vi "Insert CRC.vi"(8 "error in (no error)":errorcluster, 9 "Recalculate CRC?":bool, 10 "Frame Infos":T1 {"CRC Index" min=-7 max=7; "DLC Length  Corruption Index" min=-8 max=8}, 11 "CAN frame in":T3 {"payload" format="%x"; "timestamp" format="%<%.7X\n%x>T"; "type" items=["CAN Data"=0, "CAN Remote"=1, "CAN Bus Error"=2, "CAN 2.0 Data"=8, "CAN FD Data"=16, "CAN FD+BRS Data"=24, "J1939 Data"=192, "Delay"=224, "Log Trigger"=225, "Start Trigger"=226]; "identifier" format="%x"}) -> (0 "error out":errorcluster, 3 "CAN frame out":T3 {"payload" format="%x"; "timestamp" format="%<%.7X\n%x>T"; "type" items=["CAN Data"=0, "CAN Remote"=1, "CAN Bus Error"=2, "CAN 2.0 Data"=8, "CAN FD Data"=16, "CAN FD+BRS Data"=24, "J1939 Data"=192, "Delay"=224, "Log Trigger"=225, "Start Trigger"=226]; "identifier" format="%x"})   [LabVIEW 2018, in "CAN Gateway Engine.lvlib"]
uses:
  CAN Gateway Engine.lvlib
  <vilib>/xnet/xnet.llb/XNET Frame CAN.ctl
  <vilib>/xnet/xnet.llb/XNET Frame Type CAN.ctl
  Shared/CTLs/Frame.ctl
  Shared/CTLs/Signal_Data_Trigger.ctl
  Shared/CAN Gateway Shared.lvlib
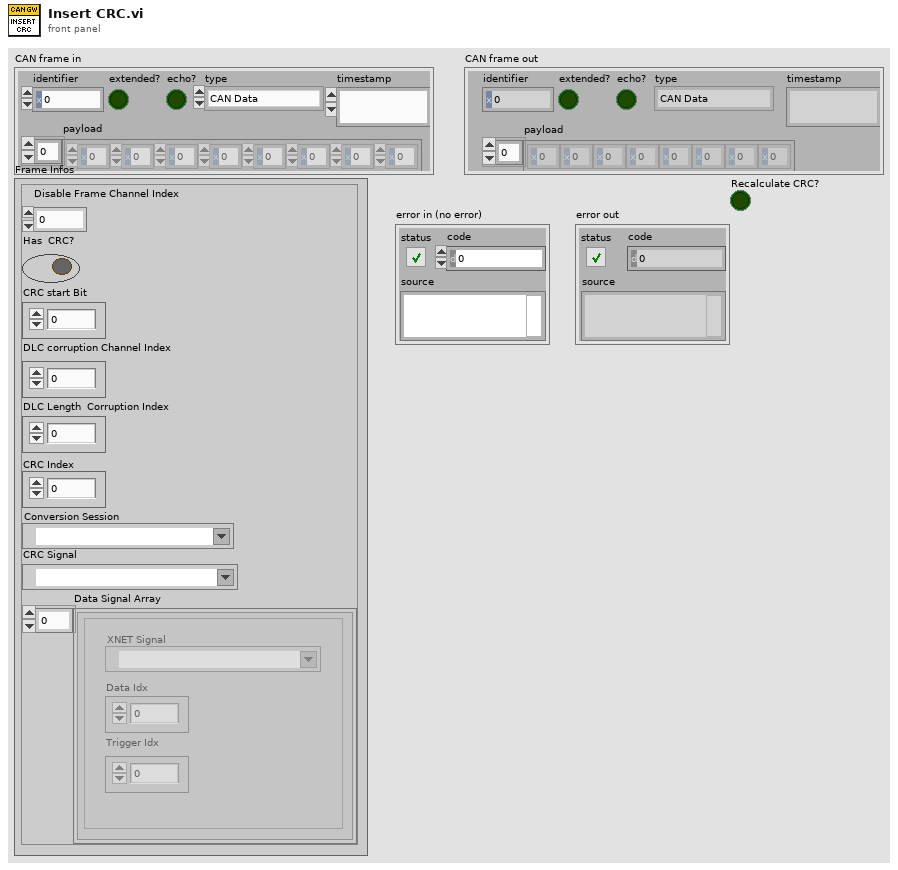
[diagram p1: front panel]
types:
  T1 = typedef "CAN Gateway Shared.lvlib/Frame.ctl" = cluster{"Disable Frame Channel Index":i32, "Has  CRC?":bool, "CRC start Bit":u32, "DLC corruption Channel Index":i32, "DLC Length  Corruption Index":i32, "CRC Index":i32, "Conversion Session":refnum<k21>, "CRC Signal":refnum<k21>, "Data Signal Array":T2[]}
  T2 = typedef "CAN Gateway Shared.lvlib/Signal_Data_Trigger.ctl" = cluster{"XNET Signal":refnum<k21>, "Data Idx":u32, "Trigger Idx":u32}
  T3 = typedef "XNET Frame CAN.ctl" = cluster{"timestamp":timestamp, "payload":u8[], "identifier":u32, "type":T4, "extended?":bool, "echo?":bool}
  T4 = typedef "XNET Frame Type CAN.ctl" = u8
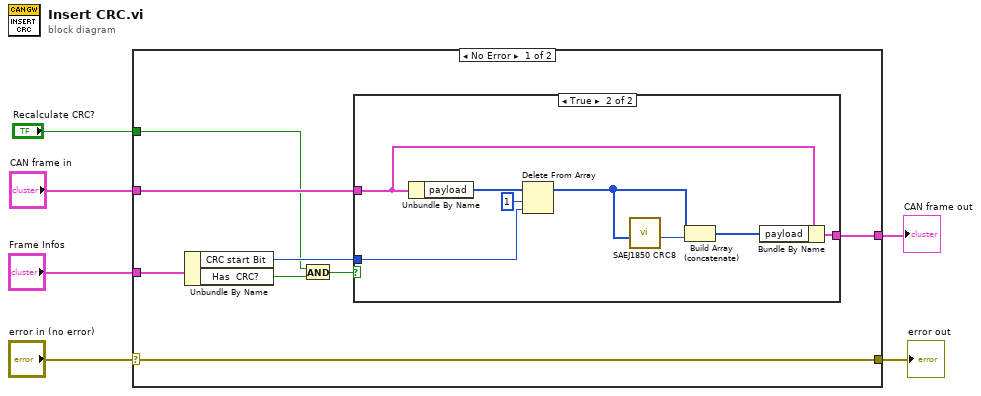
[diagram p0: block diagram]
diagram:
  n1 = case shown="No Error" "error in (no error)" {
    selector: "error in (no error)" -> [w10 w24]
    tunnel: [w14 w25] -> w6
    tunnel: "CAN frame in" -> [w12 w25]
    tunnel: "Frame Infos" -> [w11 _]
    tunnel: [w10 w24] -> w2
    tunnel: "Recalculate CRC?" -> [w9 _]
    frame No Error {
      n2 = Unbundle By Name(w11) -> ("CRC start Bit"=w13:u32, "Has  CRC?"=w8:bool)
      n3 = And(x=w9, y=w8) -> (x .and. y?=w7:bool)
      n4 = case shown="True" w7 {
        tunnel: [w15 w18] -> w14
        tunnel: w13 -> [_ w17]
        tunnel: w12 -> [w15 w16]
        frame False {
        }
        frame True {
          n5 = Unbundle By Name(w16) -> ("payload"=w23:u8[])
          n6 = Delete From Array(array=w23, length=1, index=w17) -> (array with subset deleted=w21:u8[])  [unwired: 1 out]
          n7 = call "SAEJ1850 CRC8.vi"("payload"=w21) -> ("CRC"=w20:u8)  [unwired: 10 in]
          n8 = Build Array (concatenate)(w21, w20) -> (w19:u8[])
          n9 = Bundle By Name(cluster=w16, "payload"=w19) -> (w18:T3)
        }
      }
    }
    frame Error {
    }
  }
  "CAN frame out" <- w6
  "error out" <- w2
